vi "supressDialogWindow.vi"(11 "SuppressDialogs":bool=TRUE) -> ()   [LabVIEW 2015]
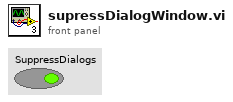
[diagram p1: front panel]
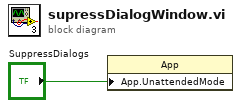
[diagram p0: block diagram]
diagram:
  n1 = property class="App"("App.UnattendedMode"="SuppressDialogs") -> ()  [unwired: 2 in, 2 out]
